vi "FestoCPX.Station.Prod.DropOK.vi"(7 "prev status":T1=enum."Error", 8 "error in":errorcluster, 10 "Serial":i32, 11 "Slot":T3) -> (0 "error out":errorcluster, 1 "Pause status":T2, 2 "Final status":T1)   [LabVIEW 2016]
uses:
  Station/Station.ProductSlot.ctl
  Sequence/Sequence.Step.Status.ctl
  Sequence/Sequence.Test.BreakReason.ctl
  tools/Translator/Translator.Message.ctl
  tools/EventLog/EventLog.EventSource.ctl
  Station/Station.ValvePosition.ctl
  tools/EventLog/EventLog.CreateError(single).vi
  tools/EventLog/EventLog.New(array).vi
  Sequence/Sequence.SerialsFglb.Action.ctl
  Sequence/Sequence.SerialsFglb.SerialData.ctl
  Global/ApplicationGlobal.vi
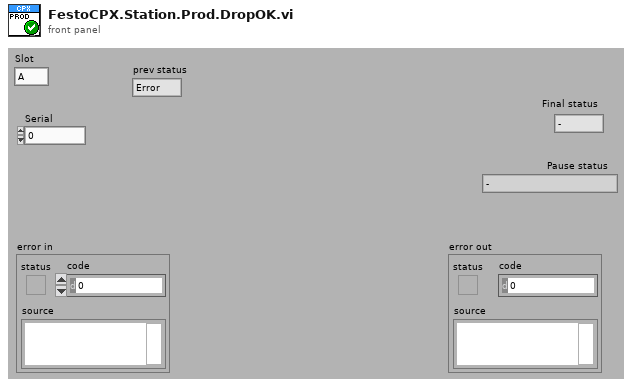
[diagram p1: front panel]
types:
  T1 = typedef "Sequence.Step.Status.ctl" = enum16{"-", "Pending", "Running", "Skipped", "Passed", "Failed", "Done", "Error", "Aborted", "Stopped"}
  T2 = typedef "Sequence.Test.BreakReason.ctl" = enum16{"-", "NOK container", "OK container", "Rev empty", "Rev missing", "Rev wrong", "Fork missing", "Fork wrong", "NOK limit", "Unload failure", "Single slot", "Part done", "Err: Prod move work", "Err: Prod move home", "Err: Prod lift work", "Err: Prod lift home", "Err: Prod Arm Work", "Err: Prod Arm NOK", "Err: Prod Arm OK", "Err: Prod NOK suck", "Err: Prod NOK drop", "Err: Prod OK missing", "Err: Prod OK suck", "Err: Prod OK drop"}
  T3 = typedef "Station.ProductSlot.ctl" = enum8{"A", "B"}
  T4 = typedef "Station.ValvePosition.ctl" = enum16{"Home", "Work"}
  T5 = typedef "Translator.Message.ctl" = enum16{"-", "Event confirmed", "Log out", "Log in", "Shutdown", "Cancel", "Start", "Begin time", "End time", "Duration", "Service Mode", "Ignore Results", "Serial Format", "On", "Off", "OK", "NOK", "NOK %s", "Home", "Work", "Close", "Open", "In progress...", "Missing", "Empty", "Hardware failure", "Initial", "Default", "Total", "Out of range", "Free disk space is below 1GB - contact technician", "Error %d >> %s", "Error %d >> %s >> %s", "Msg %d >> %s", "Laser msg %d %s", "Laser cmd error %s %d", "Laser cmd failed %s", "Laser cmd warning %s", "Laser disconnected", "Laser status %s", "Laser already started", "Laser job unkonwn %s", "Laser job missing %s", "Laser job select failure %s", "Unable to start laser printing (%s)", "Unable to stop laser printing (%s)", "Laser marking aborted", "Laser marking timeout", "Unable to reset Laser Interlock (%s)", "Unable to trigger Laser. Laser not ready (%s)", "Laser job '%s' coordinates not configured", "Starting %s", "Quitting %s", "Configured", "Initializing", "Quitting", "Loading", "Loaded %d results", "Loaded %d events", "Running", "Stopped", "Summary", "Laser", "Do you want to continue?", "Do you want to delete the configuration?", "The configuration is being used by an order. Unable to delete!", "Press confirm button", "Station is not based. Do you want to exit?", "Station requires changeover. Do you want to run the test?", "Test options are not set as default. Do you want to continue?", "Formatting of WabcoNo is disabled. Do you want to continue?", "Product not detected. Do you want to continue?", "Product scan failed. Do you want to continue?", "Calibration", "Log out?", "System", "All", "IDLE", "Translating...%s", "Not found", "Alarm %s", "Run", "Skip", "Abort", "Repeat", "Please wait...", "Database disconnected", "Database disconnected - changeover disabled!", "Login to database successful", "Login to database failed: %d; %s", "Unable to check the product status of reference %d - database disconnected", "Unable to set the product status of reference %d - database disconnected", "Variant file backup %s", "Read variant (%s)", "Result", "Station armed!", "Station requires changeover!", "Select reference number...", "EMERGENCY BUTTON - press Control button", "EMERGENCY DOOR - press Control button", "Resetting Emergency...", "Unable to reset safety circuit - Emergency Button pressed", "Unable to reset safety circuit - Emergency Side Door open", "Station not based", "Station based", "Station not empty", "Station basing...", "No order", "Press Start to begin new order", "Scanning new order", "Order NOK. Correct or scan again", "Order OK. Press Accept", "Order ready", "Revolver incorrect", "Fork incorrect", "Revolver missing", "Revolver empty", "Container missing", "Offline results", "Offline statistics", "Updating statistics %.1f %%", "DMC Configurator", "Door open", "Close the front door", "Press start button", "Done. Open the front door", "Running...", "Running...%.1f %%", "Pause %s", "Pause %s. NOK container missing", "Pause %s. OK container missing", "Pause %s. Revolver empty", "Pause %s. Revolver missing", "Pause %s. Revolver incorrect", "Pause %s. Fork missing", "Pause %s. Fork incorrect", "Pause %s. Too many failures", "Pause %s. Unloading failure", "Pause %s. One slot is not working", "Pause %s. Part order is done. Empty OK container", "Pause %s. Unable to move product to slot", "Pause %s. Unable to move back product pusher", "Pause %s. Unable to lift product", "Pause %s. Unable to move back product lifter", "Pause %s. Unable to move product arm to Work", "Pause %s. Unable to move product arm to NOK", "Pause %s. Unable to move product arm to OK", "Pause %s. Unable to unsuck the NOK product", "Pause %s. Unable to drop the NOK product", "Pause %s. Product OK missing", "Pause %s. Unable to unsuck the OK product", "Pause %s. Unable to drop the OK product", "Stopping...", "File '%s' is missing", "File '%s' is broken", "File '%s' is running", "Log file started (%s)", "Log file ended (%s)", "Log file stopped (%s)", "Log file ignored (%s)", "Log file exported (%s)", "Log file export failed (%s)", "Wrong serial number in log file", "Wrong reference number in log file", "Test steps are missing", "%s = %.3f", "Process param '%s' not found in DB", "Process param '%s' wrong order", "Process param '%s' value %.3f out of limits (%.3f; %.3f)", "Step%d param '%s' not found in DB", "Step%d param '%s' wrong order", "Step%d param '%s' value %.3f out of limits (%.3f; %.3f)", "Step%d EV '%s' not found in DB", "Step%d EV '%s' wrong order", "\"%s\" not found in DB", "\"%s\" wrong order", "\"%s\" value %.3f out of limits (%.3f; %.3f)", "\"%s\" not found in software", "Process init (%s)", "Process started", "Process restarted", "Process run", "Process done", "Process done - remove OK container", "Process aborted", "Process aborted at work", "Process aborted at home", "Process error", "Process error at home", "Process error at work", "Process close", "Process pause", "Process continue", "Process door open", "Process door close", "Process pause at slot %s due to %s", "Select plate from the order to process", "Do you want to start the process?", "Do you want to continue the process?", "There is unfinished order. Do you want to put the new order?", "Product %s %d OK", "Product %s %d NOK", "Unable to unload the slot %s. Product missing in the slot", "Unable to unload the slot %s. Product already in the arm", "Unable to accept the product as OK. Product missing in slot %s", "Unable to accept the product as OK. Product could not drop into the container at slot %s", "Unable to accept the product as NOK. Product could not drop into the container at slot %s", "Scan failed. Error %s", "Scan failed. Scanner disconnected", "Scan failed. Wrong Wabco number %d, limit (%d,%d)", "Scan failed. Wrong serial number %d, limit (%d,%d)", "Scan failed. Wrong date %d, limit (%d,%d)", "Scan failed. Wrong product wabco number %d (expected %d)", "Scan failed. Wrong product serial number %d (expected > 0)", "Scan OK %s", "Scan failed. Unable to determine table position (%s)", "Scan failed. Timeout", "Tune failed. Scanner disconnected", "Tune failed. Timeout", "%s = %d", "%s = %d->%d", "Unable to set %s = %.2f - Air Pressure Inside off", "Unable to set digital output '%s' = %d", "Unable to activate air pressure inside - timeout", "Unable to activate air pressure inside - aborted", "Unable to switch on Air Main Valve - Air Pressure Inlet off", "Unable to switch on Air Main Valve - Door open", "Unable to switch off Air Main Valve - timeout", "Unable to switch off Air Main Valve - aborted", "Unable to rotate Table - timeout", "Unable to rotate Table - aborted", "Unable to rotate Table - Product Move not in Home position", "Unable to rotate Table - Air Pressure Inside off", "Unable to rotate Table - Product Lift A not in Home position", "Unable to rotate Table - Product Lift B not in Home position", "Unable to rotate Table - unlock before movement timeout", "Unable to rotate Table - lock after movement timeout", "Unable to move Table Lock to %s position - timeout", "Unable to move Table Lock to %s position - aborted", "Unable to move Table Lock to %s position - Air Pressure Inside off", "Unable to move Table Lock to %s position - Table not in position", "Unable to move Product Lift A to %s position - timeout", "Unable to move Product Lift B to %s position - timeout", "Unable to move Product Lift A to %s position - aborted", "Unable to move Product Lift B to %s position - aborted", "Unable to move Product Lift A to %s position - Air Pressure Inside off", "Unable to move Product Lift B to %s position - Air Pressure Inside off", "Unable to move Product Lift A to %s position - Table not locked", "Unable to move Product Lift B to %s position - Table not locked", "Unable to move Product Lift A to %s position - Product Arm not in Work position", "Unable to move Product Lift B to %s position - Product Arm not in Work position", "Unable to set Product Suction Gripper %s to %s - timeout", "Unable to set Product Suction Gripper %s to %s - aborted", "Unable to set Product Suction Gripper %s to %s - Air Pressure Inside off", "Unable to set Product Suction Gripper %s to %s - Table slot unkown", "Unable to move Product Arm to %s position - timeout", "Unable to move Product Arm to %s position - aborted", "Unable to move Product Arm to %s position - Air Pressure Inside off", "Unable to move Product Arm to %s position - Product Lift A not in Home position", "Unable to move Product Arm to %s position - Product Lift B not in Home position", "Unable to move Product to %s position - timeout", "Unable to move Product to %s position - aborted", "Unable to move Product to %s position - Air Pressure Inside off", "Unable to move Product to %s position - Table not in position"}
  T6 = typedef "EventLog.EventSource.ctl" = enum16{"All", "Gui", "Ref", "File", "Arch", "Seq", "CPX", "DB", "Laser", "Scan.P", "Scan.O"}
  T7 = typedef "FestoCPX.Station.ProdPresent.ctl" = cluster{"Slot1":cluster{"A":bool, "B":bool}, "Slot2":cluster{"A":bool, "B":bool}, "Slot3":cluster{"A":bool, "B":bool}, "Slot4":cluster{"A":bool, "B":bool}, "Final":cluster{"A":bool, "B":bool}, "OK":cluster{"A":bool, "B":bool}, "Container":cluster{"OK":bool, "NOK":bool}}
  T8 = typedef "Sequence.SerialsFglb.Action.ctl" = enum16{"init", "get", "get next", "pass", "fail", "confirm", "clean"}
  T9 = typedef "Sequence.SerialsFglb.SerialData.ctl" = cluster{"TS":timestamp, "Slot":T3, "Serial":i32, "Global":bool}
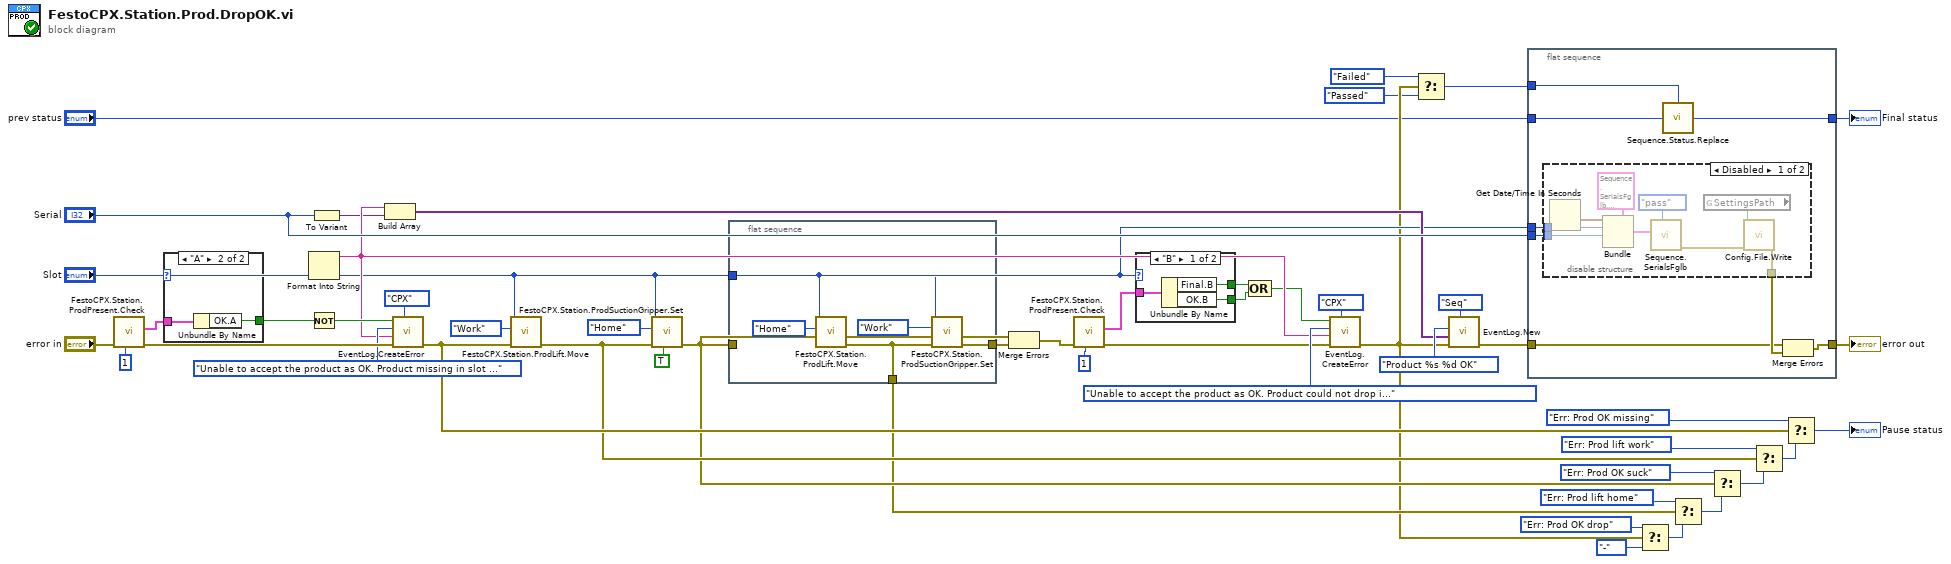
[diagram p0: block diagram]
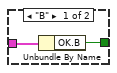
[diagram p3: hidden frame]
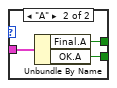
[diagram p4: hidden frame]
diagram:
  n1 = call "FestoCPX.Station.ProdPresent.Check.vi"("Stab Counter (0)"=1 ("Max Stab time [ms] (0)"), "error in"="error in") -> ("error out"=w48:errorcluster, "Prod Present"=w10:T7)  [unwired: 4 in, 4 out]
  n2 = case shown="\"A\"" "Slot" {
    tunnel: w10 -> [w53 w55]
    tunnel: [w52 w54] -> w47
    frame "B" {
      n3 = Unbundle By Name(w53) -> ("OK.B"=w52:bool)
    }
    frame "A" {
      n4 = Unbundle By Name(w55) -> ("OK.A"=w54:bool)
    }
  }
  n5 = Format Into String("Slot") -> (resulting string=w35:string)  [unwired: 3 in, 1 out]
  n6 = Not(x=w47) -> (.not. x?=w46:bool)
  n7 = To Variant(anything="Serial") -> (Variant=w34:variant)
  n8 = Build Array(w35, w34) -> (w36:variant[])
  n9 = call-poly "EventLog.CreateError.vi"("Source (All)"=EventLog.EventSource."CPX", "error in"=w48, "arg"=w35, "msg"=Translator.Message."Unable to accept the product as OK. Product missing in slot %s", "create (T)"=w46) -> ("error out"=w26:errorcluster)  [unwired: 6 in]
  n10 = call "FestoCPX.Station.ProdLift.Move.vi"("error in"=w26, "Position"=Station.ValvePosition."Work", "Slot"="Slot") -> ("error out"=w11:errorcluster)  [unwired: 8 in]
  n11 = call "FestoCPX.Station.ProdSuctionGripper.Set.vi"("wait for product (F)"=TRUE, "error in"=w11, "Position"=Station.ValvePosition."Home", "Slot"="Slot") -> ("error out"=w8:errorcluster)  [unwired: 6 in, 1 out]
  n12 = flat-sequence {
    tunnel: "Slot" -> [w56]
    tunnel: [w58] -> w14
    tunnel: w8 -> [_]
    tunnel: [w57] -> w7
    frame #0 {
      n13 = call "FestoCPX.Station.ProdLift.Move.vi"("Position"=Station.ValvePosition."Home", "Slot"=w56) -> ("error out"=w57:errorcluster)  [unwired: 9 in]
      n14 = call "FestoCPX.Station.ProdSuctionGripper.Set.vi"("error in"=w57, "Position"=Station.ValvePosition."Work", "Slot"=w56) -> ("error out"=w58:errorcluster)  [unwired: 7 in, 1 out]
    }
  }
  n15 = Merge Errors(w8, w14) -> (w6:errorcluster)
  n16 = call "FestoCPX.Station.ProdPresent.Check.vi"("Stab Counter (0)"=1 ("Max Stab time [ms] (0)"), "error in"=w6) -> ("error out"=w40:errorcluster, "Prod Present"=w43:T7)  [unwired: 4 in, 4 out]
  n17 = case shown="\"B\"" "Slot" {
    tunnel: w43 -> [w63 w66]
    tunnel: [w62 w65] -> w25
    tunnel: [w61 w64] -> w42
    frame "B" {
      n18 = Unbundle By Name(w63) -> ("Final.B"=w61:bool, "OK.B"=w62:bool)
    }
    frame "A" {
      n19 = Unbundle By Name(w66) -> ("Final.A"=w64:bool, "OK.A"=w65:bool)
    }
  }
  n20 = Compound Arithmetic op=OR(w42, w25) -> (w23:bool)
  n21 = call-poly "EventLog.CreateError.vi"("Source (All)"=EventLog.EventSource."CPX", "error in"=w40, "arg"=w35, "msg"=Translator.Message."Unable to accept the product as OK. Product could not drop into the container at slot %s", "create (T)"=w23) -> ("error out"=w5:errorcluster)  [unwired: 6 in]
  n22 = Select(t=Sequence.Step.Status."Failed", s=w5, f=Sequence.Step.Status."Passed" ("t")) -> (s? t:f=w2:T1)
  n23 = call-poly "EventLog.New.vi"("Source (All)"=EventLog.EventSource."Seq", "error in (no error)"=w5, "Arguments"=w36, "Message (-)"=Translator.Message."Product %s %d OK" ("msg")) -> ("error out"=w21:errorcluster)  [unwired: 6 in, 1 out]
  n24 = flat-sequence {
    tunnel: "Slot" -> [w74]
    tunnel: "Serial" -> [w73]
    tunnel: [w68] -> w22
    tunnel: w21 -> [w70]
    tunnel: [w72] -> w20
    tunnel: "prev status" -> [w69]
    tunnel: w2 -> [w67]
    frame #0 {
      n25 = disable-structure shown="Disabled" {
        disable-tunnel: w74 -> [w83 _]
        disable-tunnel: w73 -> [w82 _]
        disable-tunnel: [w79 _] -> w71
        frame Disabled {
          n26 = Get Date/Time In Seconds() -> (seconds since 1Jan1904=w78:timestamp)
          n27 = Bundle(cluster=T9 {"TS"=timestamp(0 s since 1904-01-01), "Slot"=enum."A", "Serial"=0, "Global"=FALSE} ("SerialData"), "TS"=w78, "Slot"=w83, "Serial"=w82) -> (w76:T9)  [unwired: 1 in]
          n28 = call "Sequence.SerialsFglb.vi"("Action (get)"=Sequence.SerialsFglb.Action."pass" ("Action"), "Serial data in"=w76) -> ("error out"=w80:errorcluster)  [unwired: 5 in, 4 out]
          n29 = global read "ApplicationGlobal.vi" "SettingsPath"() -> (w81:path)
          n30 = call "Config.File.Write.vi"("error in"=w80, "path"=w81) -> ("error out"=w79:errorcluster)  [unwired: 9 in]
        }
        frame Enabled {
        }
      }
      n31 = call "Sequence.Status.Replace.vi"("old status"=w69, "new status (Done)"=w67) -> ("status out"=w68:T1)
      n32 = Merge Errors(w70, w71) -> (w72:errorcluster)
    }
  }
  n33 = Select(t=Sequence.Test.BreakReason."Err: Prod OK drop" ("A.pause"), s=w5, f=Sequence.Test.BreakReason."-") -> (s? t:f=w18:T2)
  n34 = Select(t=Sequence.Test.BreakReason."Err: Prod lift home" ("A.pause"), s=w7, f=w18) -> (s? t:f=w17:T2)
  n35 = Select(t=Sequence.Test.BreakReason."Err: Prod OK suck" ("A.pause"), s=w8, f=w17) -> (s? t:f=w29:T2)
  n36 = Select(t=Sequence.Test.BreakReason."Err: Prod lift work" ("A.pause"), s=w11, f=w29) -> (s? t:f=w32:T2)
  n37 = Select(t=Sequence.Test.BreakReason."Err: Prod OK missing" ("A.pause"), s=w26, f=w32) -> (s? t:f=→"Pause status":T2)
  "error out" <- w20
  "Final status" <- w22
